vi "Color Segmentation.vi"() -> ()   [LabVIEW 2014]
doc: "Demonstrates how to use the IMAQ Color Segmentation function to produce a segmented greyscale image where each color, defined in a color classifier file, has a unique greyscale value in the segmented image."
uses:
  <vilib>/vision/NI_Vision_Development_Module.lvlib
panel:
  out "Color Image":T1(plugin-control)
  out "Segmented Image":T1(plugin-control)
  # "Overview: Demonstrates how to use the IMAQ Color Segmentation function to produce a segmented greyscale image where each color, defined in a color classifier file, has a unique greyscale value in the segmented image.\nRequirements: Vision Development Software.\nInstructions: Run the VI."
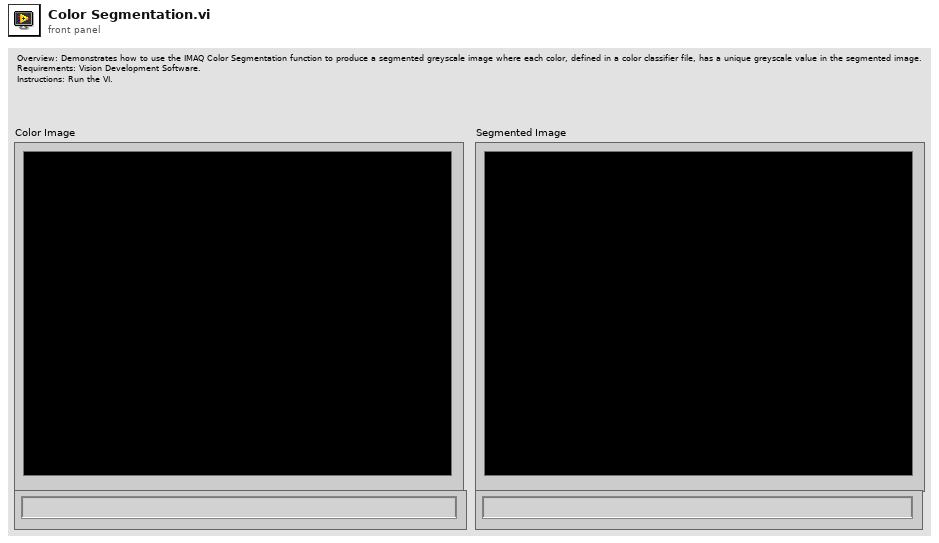
[diagram p1: front panel]
types:
  T1 = typedef "IMAQ Image.ctl" = refnum<image>
  T2 = typedef "IMAQ Rectangle" = cluster{"Left":i32, "Top":i32, "Right":i32, "Bottom":i32, "Rotation":dbl}
  T3 = typedef "Image Type" = u32
  T4 = cluster{"Window Size":cluster{"X":u32, "Y":u32}, "Step Size":u32, "Min Particle Area":u32, "Max Particle Area":u32, "Refine Segmentation?":bool}
  T5 = typedef "IMAQ Classifier Session.ctl" = refnum<k1>
  T6 = typedef "ROI Descriptor" = cluster{"Global Rectangle":i32[], "Contours":cluster{"ID":enum32{"External", "Internal"}, "Type":u32, "Coordinates":i32[]}[]}
  T7 = cluster{"Desired Font (Application)":enum16{"User-specified Font", "Application Font", "System Font", "Dialog Font"}, "[User-specified Font]":cluster{"Font Name":string, "Size":i16, "Strikeout?":bool, "Italic?":bool, "Underline?":bool, "Outline?":bool, "Shadow?":bool, "Bold?":bool, "Rotation Angle":dbl}, "Horizontal Alignment":i16, "Vertical Alignment":i16}
  T8 = cluster{"Global Rectangle[0]":i32, "Global Rectangle[1]":i32}
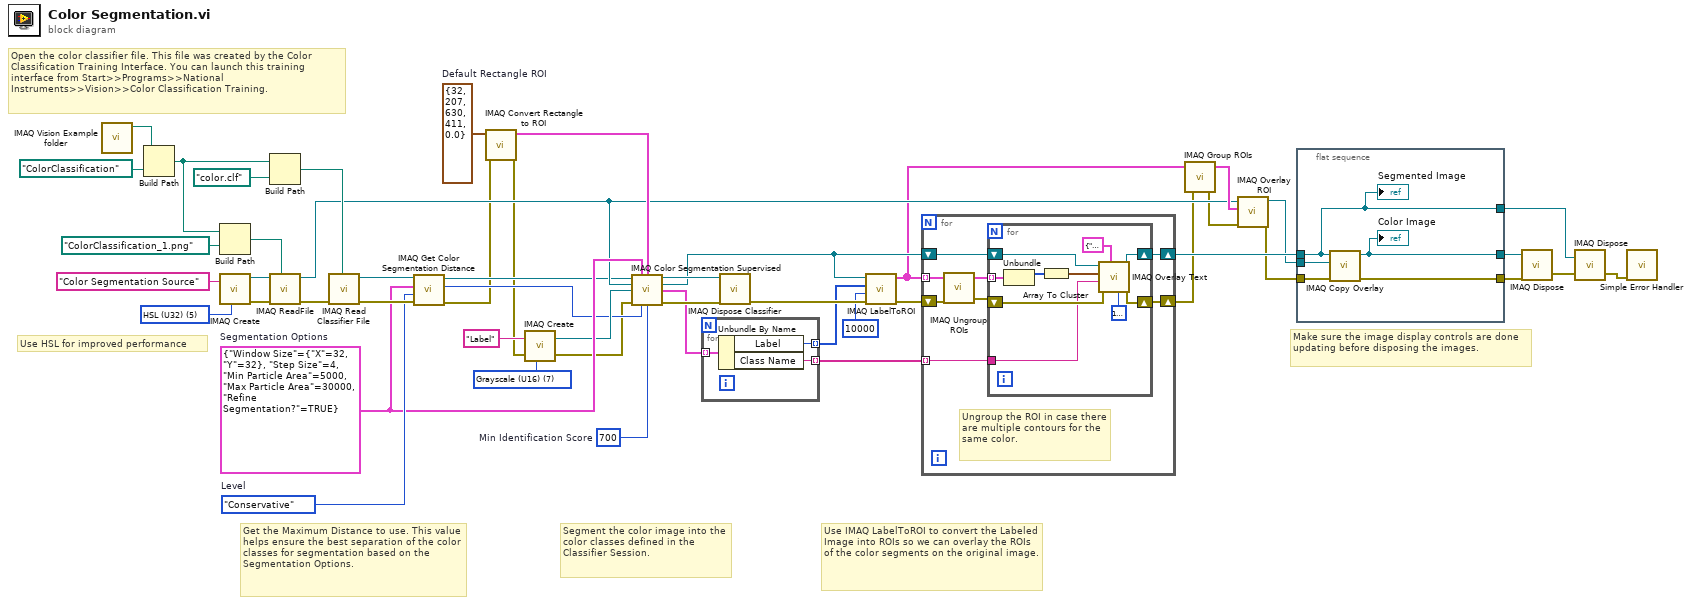
[diagram p0: block diagram]
diagram:
  w24 = T2 {"Left"=32, "Top"=207, "Right"=630, "Bottom"=411, "Rotation"=0.0}  # Default Rectangle ROI
  w29 = 700  # Min Identification Score
  w33 = enum32{"Conservative", "Aggressive"}."Conservative"  # Level
  w42 = T3 7 items=["Grayscale (U8)", "Grayscale (I16)", "Grayscale (SGL)", "Complex (CSG)", "RGB (U32)", "HSL (U32)", "RGB (U64)", "Grayscale (U16)"] ("Image Type")
  w44 = T3 5 items=["Grayscale (U8)", "Grayscale (I16)", "Grayscale (SGL)", "Complex (CSG)", "RGB (U32)", "HSL (U32)", "RGB (U64)", "Grayscale (U16)"] ("Image Type")
  w32 = T4 {"Window Size"={"X"=32, "Y"=32}, "Step Size"=4, "Min Particle Area"=5000, "Max Particle Area"=30000, "Refine Segmentation?"=TRUE}  # Segmentation Options
  # "Use HSL for improved performance"
  # "Make sure the image display controls are done updating before disposing the images."
  # "Use IMAQ LabelToROI to convert the Labeled Image into ROIs so we can overlay the ROIs of the color segments on the original image."
  # "Segment the color image into the color classes defined in the Classifier Session."
  # "Open the color classifier file. This file was created by the Color Classification Training Interface. You can launch this training interface from Start>>Programs>>National Instruments>>Vision>>Color Classification Training."
  # "Get the Maximum Distance to use. This value helps ensure the best separation of the color classes for segmentation based on the Segmentation Options."
  n1 = call "IMAQ Vision Example folder.vi"() -> ("Example Image Path"=w49:path)  [unwired: 11 in]
  n2 = Build Path(base path=w49, name or relative path=path "ColorClassification") -> (appended path=w39:path)
  n3 = Build Path(base path=w39, name or relative path=path "ColorClassification_1.png") -> (appended path=w37:path)
  n4 = call "IMAQ Create"("Image Name"="Color Segmentation Source", "Image Type"=w44) -> ("New Image"=w41:T1, "error out"=w40:errorcluster)  [unwired: 2 in, 1 out]
  n5 = Build Path(base path=w39, name or relative path=path "color.clf") -> (appended path=w45:path)
  n6 = call "IMAQ ReadFile"("File Path"=w37, "error in (no error)"=w40, "Image"=w41) -> ("error out"=w36:errorcluster, "Image Out"=w12:T1)  [unwired: 4 in, 3 out]
  n7 = call "IMAQ Read Classifier File"("File Path"=w45, "error in (no error)"=w36) -> ("error out"=w34:errorcluster, "Classifier Session"=w35:T5)  [unwired: 2 in, 6 out]
  n8 = call "IMAQ Get Color Segmentation Distance"("error in (no error)"=w34, "Level"=w33, "Segmentation Options"=w32, "Color Classifier Session"=w35) -> ("error out"=w6:errorcluster, "Maximum Distance"=w30:i32, "Color Classifier Session (dup)"=w8:T5)  [unwired: 5 in]
  n9 = call "IMAQ Convert Rectangle to ROI"("error in (no error)"=w6, "Rectangle"=w24) -> ("error out"=w3:errorcluster, "ROI Descriptor"=w23:T6)  [unwired: 7 in]
  n10 = call "IMAQ Create"("Image Name"="Label", "Image Type"=w42, "error in (no error)"=w3) -> ("New Image"=w31:T1, "error out"=w2:errorcluster)  [unwired: 1 in, 1 out]
  n11 = call "IMAQ Color Segmentation Supervised"("Color Classifier Session"=w8, "Segmentation Options"=w32, "ROI Descriptor"=w23, "Image"=w12, "Label Image"=w31, "error in (no error)"=w2, "Maximum Distance"=w30, "Min Identification Score"=w29) -> ("Color Classifier Session (dup)"=w27:T5, "Label Image Out"=w18:T1, "Labels Out"=w25:cluster{"Class Name":string, "Label":u32}[], "error out"=w28:errorcluster)  [unwired: 1 in, 3 out]
  n12 = for {
    tunnel: w25 -> [w52] mode=indexing
    tunnel: [w51] -> w22 mode=indexing
    tunnel: [w50] -> w20 mode=indexing
    n13 = Unbundle By Name(w52) -> ("Label"=w51:u32, "Class Name"=w50:string)
  }
  n14 = call "IMAQ Dispose Classifier"("error in (no error)"=w28, "Classifier Session"=w27) -> ("error out"=w26:errorcluster)  [unwired: 9 out]
  n15 = call "IMAQ LabelToROI"("error in (no error)"=w26, "Max number of vectors in ROI"=10000, "Labels In"=w22, "Image"=w18) -> ("error out"=w19:errorcluster, "ROIs"=w1:T6[])  [unwired: 1 in, 5 out]
  n16 = for {
    tunnel: w1 -> [w58] mode=indexing
    tunnel: w20 -> [w54] mode=indexing
    shift-right: [w59] -> w14
    shift-left: w18 -> [w60]
    shift-right: [w53] -> w5
    shift-left: w19 -> [w56]
    # "Ungroup the ROI in case there are multiple contours for the same color."
    n17 = call "IMAQ Ungroup ROIs"("error in (no error)"=w56, "ROI Descriptor"=w58) -> ("error out"=w55:errorcluster, "ROI Descriptors out"=w57:T6[])  [unwired: 2 in]
    n18 = for {
      tunnel: w57 -> [w64] mode=indexing
      shift-right: [w65] -> w59
      shift-left: w60 -> [w68]
      shift-right: [w62] -> w53
      shift-left: w55 -> [w63]
      tunnel: w54 -> [w61]
      n19 = Unbundle(w64) -> ("Global Rectangle"=w70:i32[])  [unwired: 1 out]
      n20 = Array To Cluster(array=w70) -> (cluster=w69:T8)
      n21 = call "IMAQ Overlay Text"("BG Color (Transparent)"=u32 16777226, "Font, Size & Style"=T7 {"Desired Font (Application)"=enum."Application Font", "[User-specified Font]"={"Font Name"="", "Size"=12, "Strikeout?"=FALSE, "Italic?"=FALSE, "Underline?"=FALSE, "Outline?"=FALSE, "Shadow?"=FALSE, "Bold?"=FALSE, "Rotation Angle"=0.0}, "Horizontal Alignment"=0, "Vertical Alignment"=1}, "error in (no error)"=w63, "String"=w61, "Origin"=w69, "Image"=w68) -> ("error out"=w62:errorcluster, "Image Out"=w65:T1)  [unwired: 4 in]
    }
  }
  n22 = call "IMAQ Group ROIs"("error in (no error)"=w5, "ROI Descriptors"=w1) -> ("error out"=w4:errorcluster, "ROI Descriptor out"=w13:T6)  [unwired: 2 in]
  n23 = call "IMAQ Overlay ROI"("error in (no error)"=w4, "ROI Descriptor"=w13, "Image"=w12) -> ("error out"=w10:errorcluster, "Image Out"=w11:T1)  [unwired: 7 in]
  n24 = flat-sequence {
    tunnel: w10 -> [w75]
    tunnel: [w74] -> w17
    tunnel: w11 -> [w73]
    tunnel: [w72] -> w16
    tunnel: w14 -> [w71]
    tunnel: [w71] -> w9
    frame #0 {
      n25 = call "IMAQ Copy Overlay"("error in (no error)"=w75, "Image Dst"=w73, "Image Src"=w71) -> ("error out"=w74:errorcluster, "Image Dst Out"=w72:T1)  [unwired: 7 in]
      "Color Image" <- w72
      "Segmented Image" <- w71
    }
  }
  n26 = call "IMAQ Dispose"("Image"=w16, "error in (no error)"=w17) -> ("error out"=w15:errorcluster)  [unwired: 1 in, 3 out]
  n27 = call "IMAQ Dispose"("Image"=w9, "error in (no error)"=w15) -> ("error out"=w7:errorcluster)  [unwired: 1 in, 3 out]
  n28 = call <vilib>:"Simple Error Handler.vi"("error in (no error)"=w7) -> ()  [unwired: 4 in, 5 out]
